vi "gwyscan refine path threshold.vi"(0 "xypos":dbl[](array[numeric]), 1 "xypos_prev":dbl[](array[numeric]), 2 "zdata_prev":dbl[](array[numeric]), 3 "n_prev":i32, 4 "channel_prev":i32, 5 "xypos_preprev":dbl[](array[numeric]), 6 "zdata_preprev":dbl[](array[numeric]), 7 "error in (no error)":errorcluster, 8 "n_preprev":i32, 9 "channel_preprev":i32, 10 "threshold":dbl, 11 "xdiv":i32, 12 "ydiv":i32, 13 "xstep":dbl, 14 "ystep":dbl, 15 "xreal":dbl, 16 "yreal":dbl, 17 "xoffset":dbl, 18 "yoffset":dbl) -> (20 "xypos OUT":dbl[](array[numeric]), 21 "xypos_prev OUT":dbl[](array[numeric]), 22 "zdata_prev OUT":dbl[](array[numeric]), 23 "xypos_preprev OUT":dbl[](array[numeric]), 24 "zdata_preprev OUT":dbl[](array[numeric]), 26 "function return":i32, 27 "error out":errorcluster)   [LabVIEW 2016, in "libgwyscan.lvlib"]
doc: "GWYSCANDLL_API int gwyscan_refine_path_threshold(double* xypos, \n const double* xypos_prev, \n const double* zdata_prev, \n int n_prev, \n int channel_prev, \n const double* xypos_preprev,\n const double* zdata_preprev, \n int n_preprev, \n int channel_preprev, \n double threshold, \n int xdiv, \n int ydiv, \n double xstep, \n double ystep, \n double xreal, \n double yreal, \n double xoffset, \n double yoffset);"
uses:
  libgwyscan.lvlib
  libgwyscan.dll
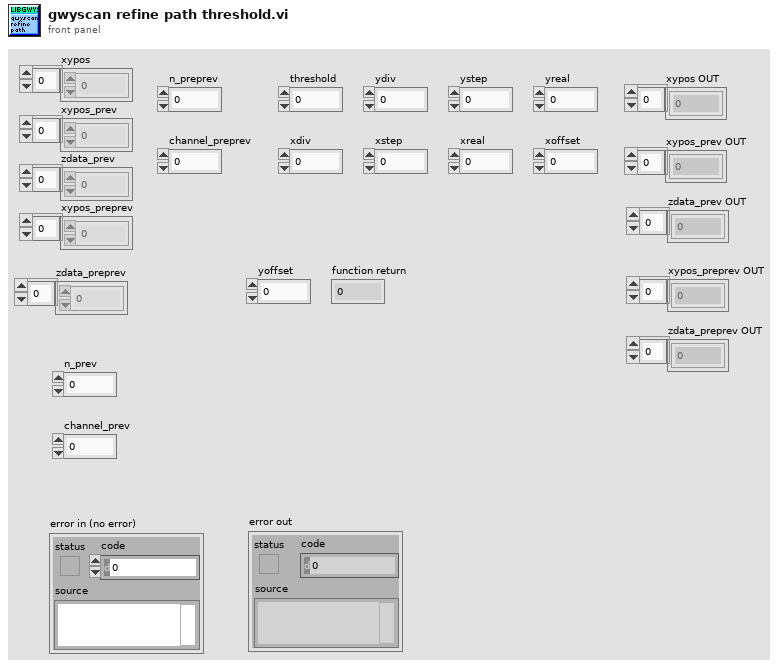
[diagram p1: front panel]
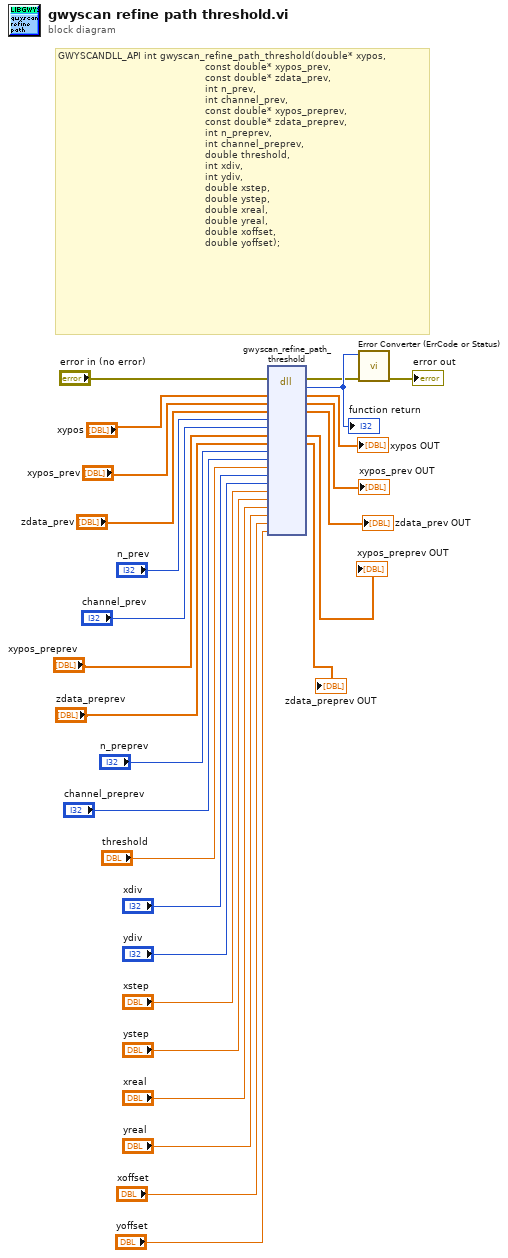
[diagram p0: block diagram]
diagram:
  # "GWYSCANDLL_API int gwyscan_refine_path_threshold(double* xypos, \n                                                 const double* xypos_prev, \n                                                 const double* zdata_prev, \n                                                 int n_prev, \n                                                 int channel_prev, \n                                                 const double* xypos_preprev,\n                                                 const double* zdata_preprev, \n                                                 int n_preprev, \n                                                 int channel_preprev, \n                                                 double threshold, \n                                                 int xdiv, \n                                                 int ydiv, \n                                                 double xstep, \n                                                 double ystep, \n                                                 double xreal, \n                                                 double yreal, \n                                                 double xoffset, \n                                                 double yoffset);"
  n1 = dll-call lib="PTH2’abs CUsersCharlÃ¨ne BrillardDesktoplbni-lbniAFMController-BetaVersionv2.0.16-20190611 libgwyscan-1.2-labview2015-win32libgwyscan.dll" fn="gwyscan_refine_path_threshold"(error in="error in (no error)", "xypos"="xypos", "xypos_prev"="xypos_prev", "zdata_prev"="zdata_prev", "n_prev"="n_prev", "channel_prev"="channel_prev", "xypos_preprev"="xypos_preprev", "zdata_preprev"="zdata_preprev", "n_preprev"="n_preprev", "channel_preprev"="channel_preprev", "threshold"="threshold", "xdiv"="xdiv", "ydiv"="ydiv", "xstep"="xstep", "ystep"="ystep", "xreal"="xreal", "yreal"="yreal", "xoffset"="xoffset", "yoffset"="yoffset") -> (error out=w7:errorcluster, "return type"=w27:i32, "xypos"=→"xypos OUT":dbl[], "xypos_prev"=→"xypos_prev OUT":dbl[], "zdata_prev"=→"zdata_prev OUT":dbl[], "xypos_preprev"=→"xypos_preprev OUT":dbl[], "zdata_preprev"=→"zdata_preprev OUT":dbl[])  [unwired: 15 in, 1 out]
  "function return" <- w27
  n2 = call "Error Converter (ErrCode or Status).vi"("error in (no error)"=w7, "error code"=w27) -> ("error out"=→"error out":errorcluster)  [unwired: 9 in]
